vi "RDS Configuration Utility.vi"() -> ()   [LabVIEW 2015, in "RDS Configuration Library.lvlib"]
uses:
  RDS Configuration Library.lvlib
  RDS Configuration.ctl
  RDS Child Messages/PID Gains/PID Gains Control.ctl
  RDS Mission Controller Actor/Mission Controller Settings.ctl
  RDS Child Messages/RDS Child Messages.lvlib
  RDS Mission Controller Actor/RDS Mission Controller Actor.lvlib
panel:
  in  "RDS Config":T1={"State Update Rate (Hz)"=0.0, "Helm Rate (Hz)"=0.0, "Helm Gains"={"P (Kc)"=0.0, "I (Ti)"=0.0, "D (Td)"=0.0}, "Limiter"=100.0, "Mission Controller Settings"={"Waypoint Radius (m)"=0.0}, "Mag Dev"=0.0} {"Helm Gains"."D (Td)" format="%#_9f"; "Helm Gains"."I (Ti)" format="%#_9f"; "Helm Gains"."P (Kc)" format="%#.9f"}
  in  "Close":bool
  in  "Read":bool
  in  "Write":bool
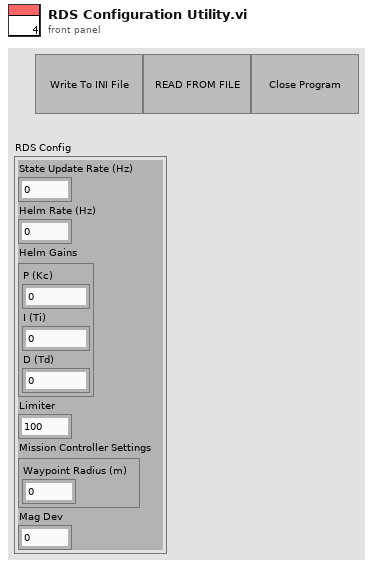
[diagram p1: front panel]
types:
  T1 = typedef "RDS Configuration Library.lvlib/RDS Configuration.ctl" = cluster{"State Update Rate (Hz)":dbl, "Helm Rate (Hz)":dbl, "Helm Gains":T2, "Limiter":dbl, "Mission Controller Settings":T3, "Mag Dev":dbl}
  T2 = typedef "RDS Child Messages.lvlib/PID Gains Control.ctl" = cluster{"P (Kc)":sgl, "I (Ti)":sgl, "D (Td)":sgl}
  T3 = typedef "RDS Mission Controller Actor.lvlib/Mission Controller Settings.ctl" = cluster{"Waypoint Radius (m)":dbl}
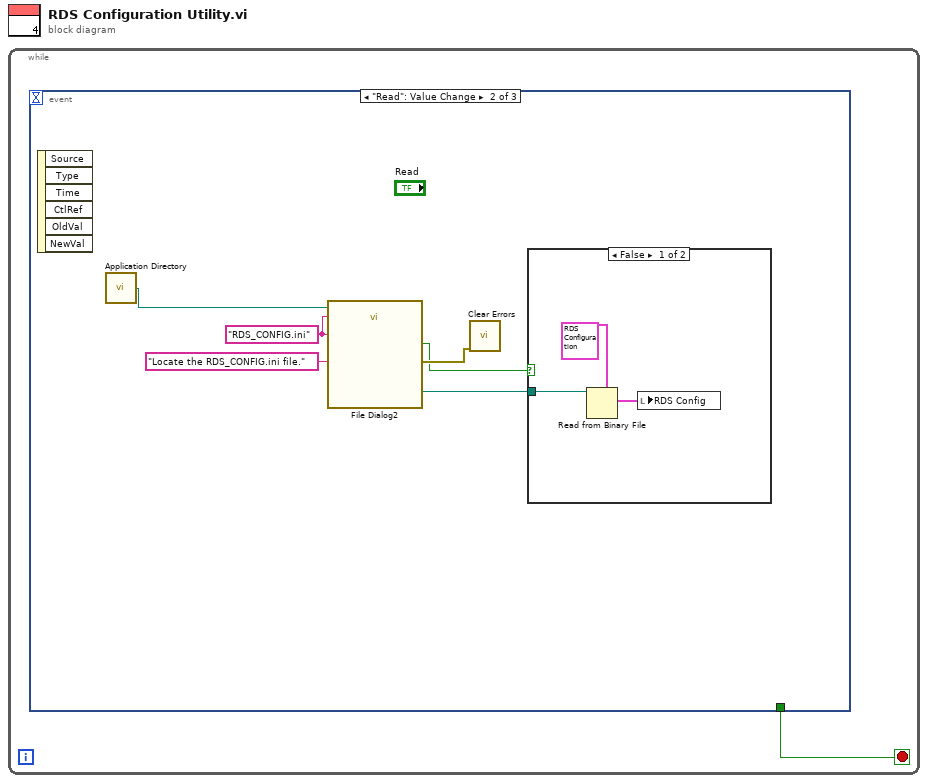
[diagram p0: block diagram]
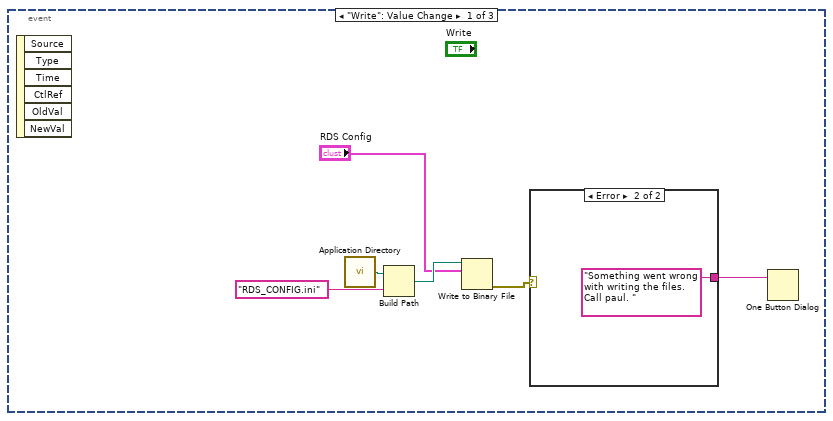
[diagram p2: hidden frame]
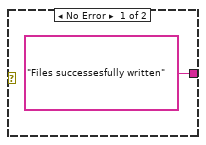
[diagram p3: hidden frame]
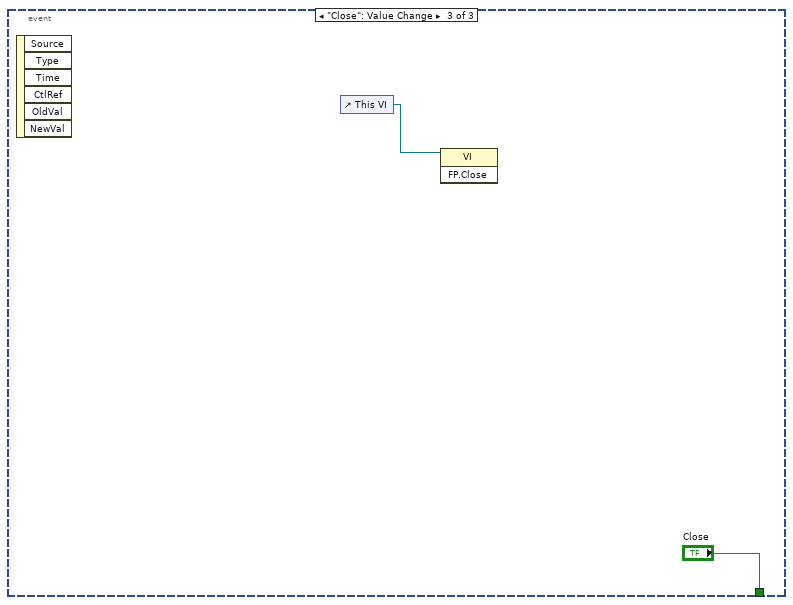
[diagram p5: hidden frame]
diagram:
  n1 = while {
    stop <- w1 stop-if-true
    n2 = event shown="[1] \"Read\": Value Change" {
      selector: _ -> [_ _ _]
      dyn-events: _ -> [_ _ _]
      timeout: _ -> [_ _ _]
      tunnel: [_ _ "Close"] -> w1
      event "Write": Value Change {
        n3 = event-data() -> ()  [unwired: 1 in, 6 out]
        n4 = call <vilib>:"Application Directory.vi"() -> ("Application Directory"=w6:path)
        n5 = Build Path(base path=w6, name or relative path="RDS_CONFIG.ini") -> (appended path=w5:path)
        n6 = Write to Binary File(file (use dialog)=w5, data="RDS Config") -> (error out=w3:errorcluster)  [unwired: 4 in, 2 out]
        n7 = case shown="Error" w3 {
          tunnel: ["Files successesfully written" "Something went wrong with writing the files. Call paul. "] -> w2
          frame No Error {
          }
          frame Error {
          }
        }
        n8 = One Button Dialog(message=w2) -> ()  [unwired: 1 in, 1 out]
      }
      event "Read": Value Change {
        w14 = "RDS_CONFIG.ini" ("pattern (all files)")
        n9 = event-data() -> ()  [unwired: 1 in, 6 out]
        n10 = call <vilib>:"Application Directory.vi"() -> ("Application Directory"=w10:path)
        n11 = call "File Dialog2"("start path"=w10, "prompt"="Locate the RDS_CONFIG.ini file.", "default name"=w14, "pattern (all files)"=w14) -> ("selected path"=w15:path, "cancelled"=w11:bool, "error out"=w12:errorcluster)  [unwired: 8 in, 1 out]
        n12 = call <vilib>:"Clear Errors.vi"("error in (no error)"=w12) -> ()  [unwired: 5 in, 2 out]
        n13 = case shown="False" w11 {
          tunnel: w15 -> [w18 _]
          frame False {
            n14 = Read from Binary File(5:T1 {"State Update Rate (Hz)"=0.0, "Helm Rate (Hz)"=0.0, "Helm Gains"={"P (Kc)"=0.0, "I (Ti)"=0.0, "D (Td)"=0.0}, "Limiter"=100.0, "Mission Controller Settings"={"Waypoint Radius (m)"=0.0}, "Mag Dev"=0.0} ("RDS Config"), 11:w18) -> (2:w16:T1)  [unwired: 4 in, 3 out]
            n15 = local write "RDS Config"(w16) -> ()
          }
          frame True {
          }
        }
      }
      event "Close": Value Change {
        n16 = event-data() -> ()  [unwired: 1 in, 6 out]
        n17 = control-ref of="This VI"() -> (w20:refnum<vi>)
        n18 = invoke class="VI" method="FP.Close"(reference=w20) -> ()  [unwired: 2 in, 3 out]
      }
    }
  }
